vi "Evaluate Menu Selection.vi"(8 "error in":errorcluster, 9 "ItemPath":string, 10 "ItemTag":string, 11 "MQ in":refnum<class "Delacor_lib_QMH_Message Queue.lvclass">) -> (0 "error out":errorcluster)   [LabVIEW 2022 SP3, in "UI Manager.lvlib"]
doc: "____\nHAMPEL SOFTWARE ENGINEERING v2.6.0 (2023-12-19 10:54)"
uses:
  UI Manager.lvlib
  <vilib>/Delacor/Delacor QMH/Libraries/Message Queue_class/Delacor_lib_QMH_Message Queue.lvclass
  Shutdown Application Argument--cluster.ctl
  <vilib>/Delacor/Delacor QMH/Libraries/Message Queue_class/Delacor_lib_QMH_Message Queue.lvclass/Delacor_lib_QMH_Message Queue.ctl
  Display another Module UI Argument--cluster.ctl
  Module Display Scenarios.ctl
  Libraries/hse-libraries/Source/hse-application/hse-application.lvclass/hse-application.ctl
  <vilib>/Delacor/Delacor QMH/Libraries/Message Queue_class/Delacor_lib_QMH_Enqueue Message (Single).vi
  Libraries/hse-libraries/Source/hse-application/HSE Application not initialized--error.vi
  <vilib>/Utility/error.llb/Clear Errors.vi
  Libraries/hse-libraries/Source/hse-application/hse-application__GetSingleton.vi
  <vilib>/Utility/sysdir.llb/Get System Directory.vi
  <vilib>/Utility/error.llb/Error Cluster From Error Code.vi
  Libraries/hse-libraries/Source/hse-application/hse-application.lvclass
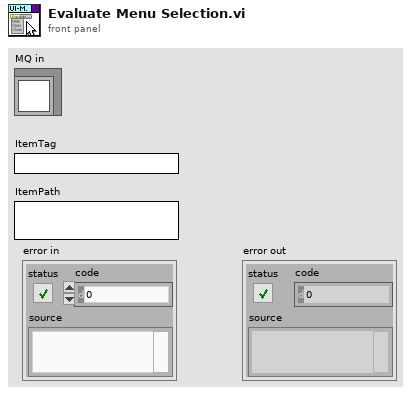
[diagram p1: front panel]
types:
  T1 = typedef "UI Manager.lvlib/Shutdown Application Argument--cluster.ctl" = cluster{"User Confirm?":bool}
  T2 = typedef "UI Manager.lvlib/Module Display Scenarios.ctl" = enum16{"Stand-Alone", "Managed"}
  T3 = typedef "UI Manager.lvlib/Display another Module UI Argument--cluster.ctl" = cluster{"Module DQMH Path":path, "Display Scenario":T2}
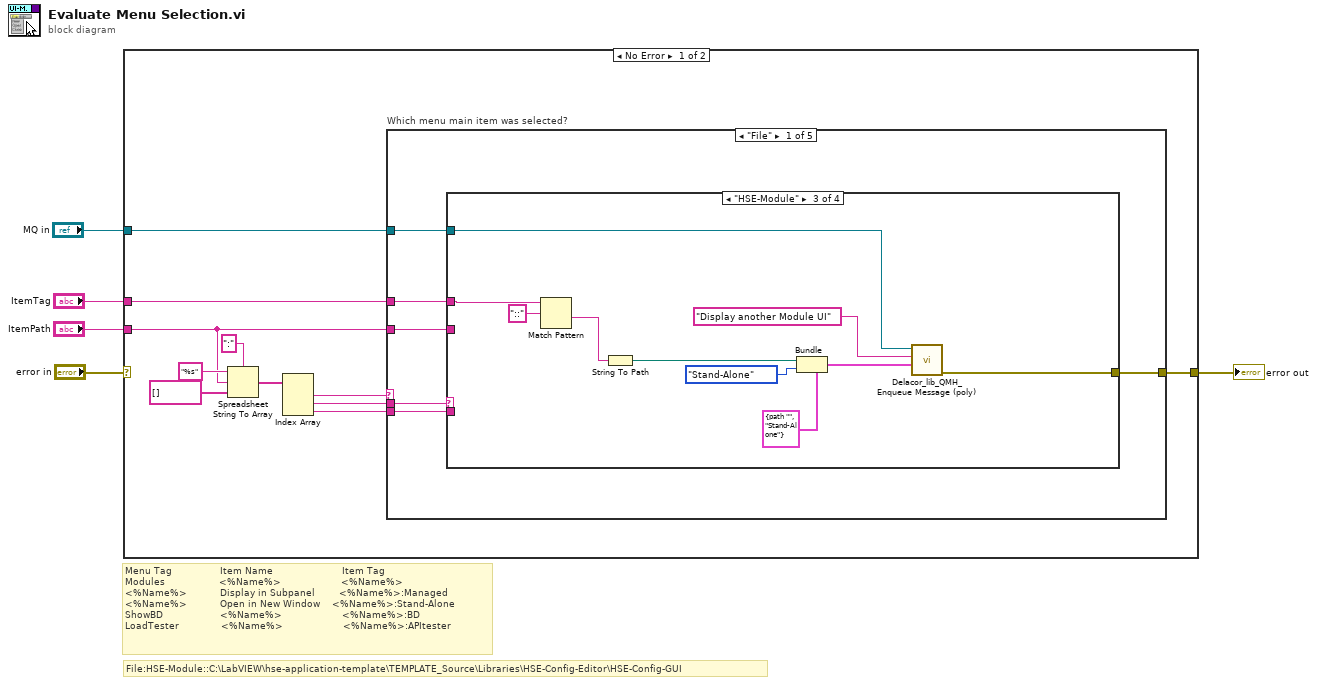
[diagram p0: block diagram]
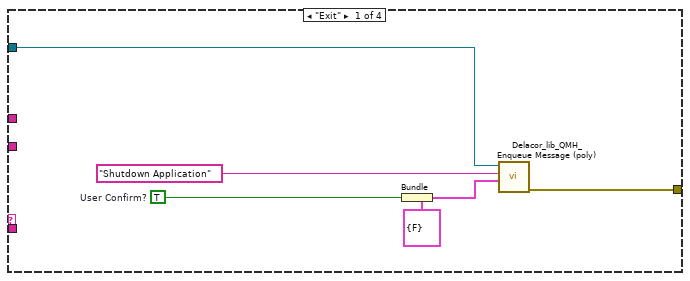
[diagram p2: hidden frame]
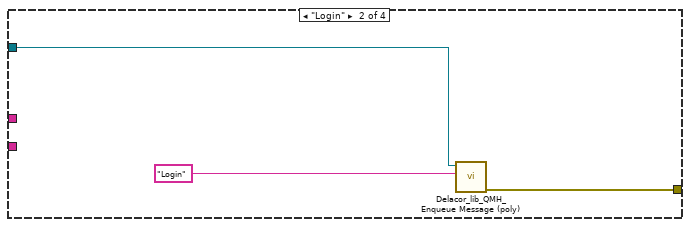
[diagram p3: hidden frame]
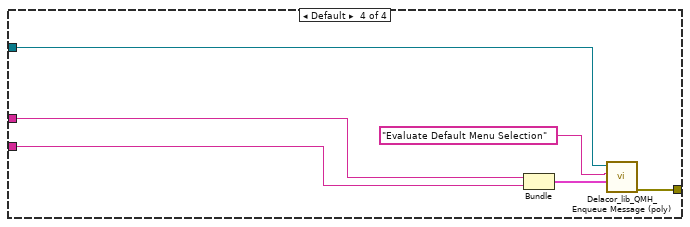
[diagram p4: hidden frame]
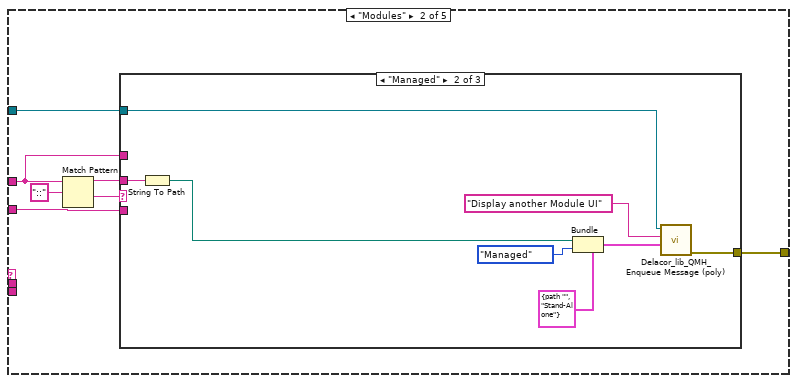
[diagram p5: hidden frame]
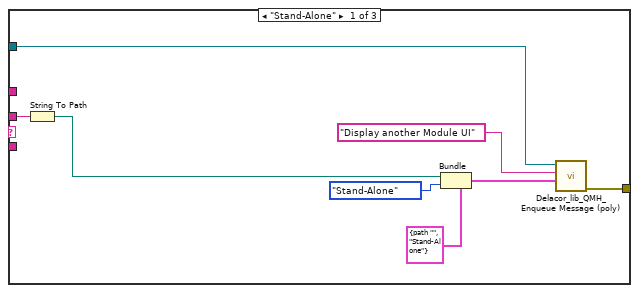
[diagram p6: hidden frame]
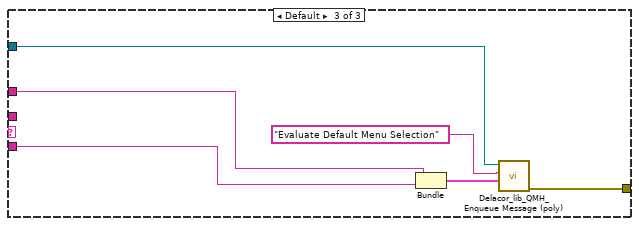
[diagram p7: hidden frame]
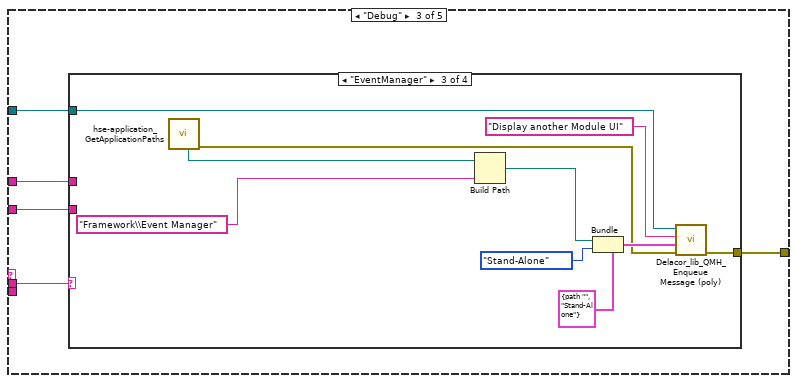
[diagram p8: hidden frame]
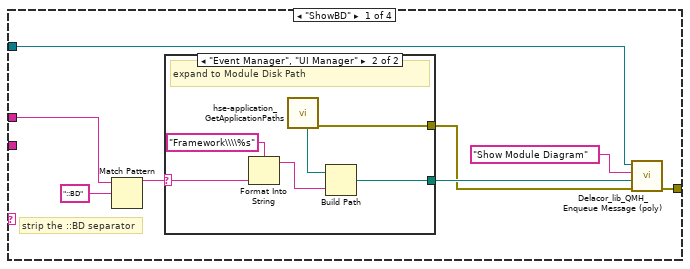
[diagram p9: hidden frame]
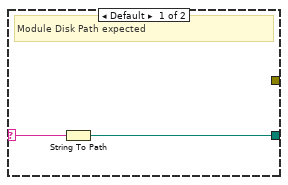
[diagram p10: hidden frame]
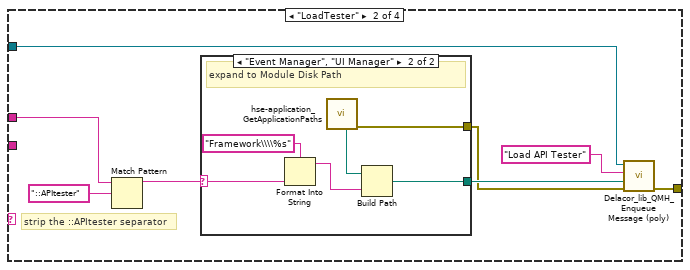
[diagram p11: hidden frame]
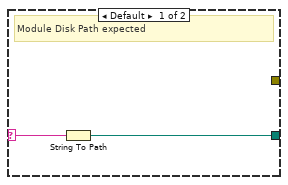
[diagram p12: hidden frame]
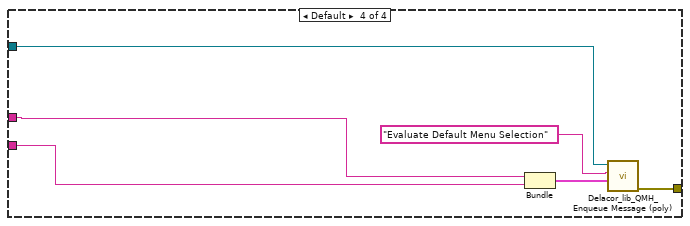
[diagram p13: hidden frame]
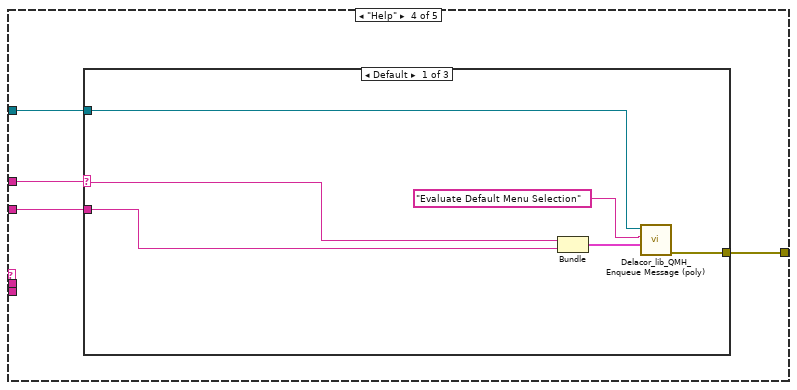
[diagram p14: hidden frame]
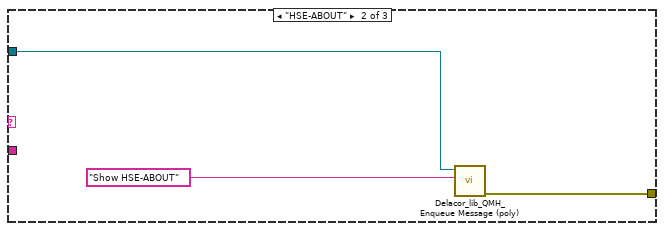
[diagram p15: hidden frame]
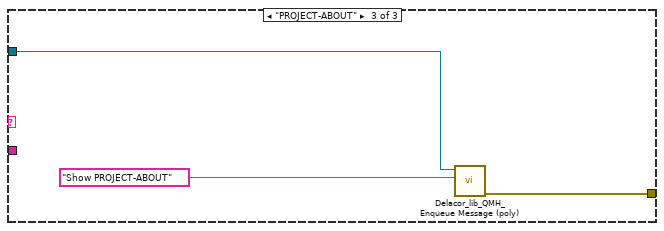
[diagram p16: hidden frame]
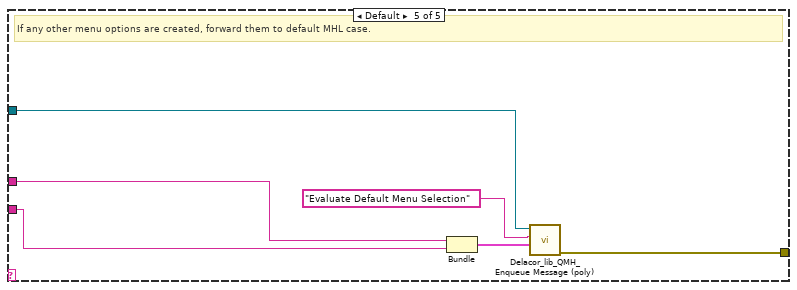
[diagram p17: hidden frame]
diagram:
  # "File:HSE-Module::C:\\LabVIEW\\hse-application-template\\TEMPLATE_Source\\Libraries\\HSE-Config-Editor\\HSE-Config-GUI"
  # "Menu Tag                Item Name\t                      Item Tag\nModules\t                 <%Name%>                   \t<%Name%>\n<%Name%>          \tDisplay in Subpanel       \t<%Name%>:Managed\n<%Name%>          \tOpen in New Window   \t<%Name%>:Stand-Alone\nShowBD                   <%Name%>\t                   <%Name%>:BD\nLoadTester\t             <%Name%>                   \t<%Name%>:APItester"
  n1 = case shown="No Error" "error in" {
    selector: "error in" -> [_ w152]
    tunnel: "ItemPath" -> [w6 _]
    tunnel: "MQ in" -> [w14 _]
    tunnel: "ItemTag" -> [w13 _]
    tunnel: [w11 w152] -> w2
    frame No Error {
      n2 = Spreadsheet String To Array(delimiter (Tab)=":", format string="%s", spreadsheet string=w6, array type (2D Dbl)=string[] []) -> (array=w10:string[])
      n3 = Index Array(array=w10) -> (element #1=w9:string, element #2=w7:string, element #3=w8:string)  [unwired: 3 in]
      n4 = case "Which menu main item was selected?" shown="\"File\"" w9 {
        tunnel: w14 -> [w22 w54 w81 w133 w151]
        tunnel: [w21 w53 w79 w132 w150] -> w11
        tunnel: w13 -> [w20 w49 w80 w131 w149]
        tunnel: w8 -> [w17 _ _ _ _]
        tunnel: w7 -> [w18 _ w78 _ _]
        tunnel: w6 -> [w19 w48 w77 w130 w146]
        frame "File" {
          n5 = case shown="\"HSE-Module\"" w18 {
            tunnel: w22 -> [w27 w30 w36 w44]
            tunnel: [w26 w29 w35 w45] -> w21
            tunnel: w19 -> [_ _ _ w42]
            tunnel: w20 -> [_ _ w33 w43]
            tunnel: w17 -> [_ _ _ _]
            frame "Exit" {
              w24 = TRUE  # User Confirm?
              n6 = Bundle(cluster=T1 {"User Confirm?"=FALSE} ("Shutdown Application Argument"), "User Confirm?"=w24) -> (w23:T1)
              n7 = call-poly <vilib>:"Delacor_lib_QMH_Enqueue Message (poly).vi"("Message Data"=w23, "Message"="Shutdown Application", "Message Queue in"=w27) -> ("error out"=w26:errorcluster)  [unwired: 7 in, 1 out]
            }
            frame "Login" {
              n8 = call-poly <vilib>:"Delacor_lib_QMH_Enqueue Message (poly).vi"("Message"="Login", "Message Queue in"=w30) -> ("error out"=w29:errorcluster)  [unwired: 8 in, 1 out]
            }
            frame "HSE-Module" {
              n9 = Match Pattern(string=w33, regular expression="::") -> (after substring=w32:string)  [unwired: 1 in, 3 out]
              n10 = String To Path(string=w32) -> (path=w41:path)
              n11 = Bundle(cluster=T3 {"Module DQMH Path"=path "", "Display Scenario"=enum."Stand-Alone"} ("Display Module UI Argument"), "Module DQMH Path"=w41, "Display Scenario"=Module_Display_Scenarios."Stand-Alone") -> (w38:T3)
              n12 = call-poly <vilib>:"Delacor_lib_QMH_Enqueue Message (poly).vi"("Message Data"=w38, "Message"="Display another Module UI", "Message Queue in"=w36) -> ("error out"=w35:errorcluster)  [unwired: 7 in, 1 out]
            }
            frame Default {
              n13 = Bundle("ItemTag"=w43, "ItemPath"=w42) -> (w46:cluster{"ItemTag":string, "ItemPath":string})  [unwired: 1 in]
              n14 = call-poly <vilib>:"Delacor_lib_QMH_Enqueue Message (poly).vi"("Message Data"=w46, "Message"="Evaluate Default Menu Selection", "Message Queue in"=w44) -> ("error out"=w45:errorcluster)  [unwired: 7 in, 1 out]
            }
          }
        }
        frame "Modules" {
          n15 = Match Pattern(string=w49, regular expression="::") -> (before substring=w50:string, after substring=w51:string)  [unwired: 1 in, 2 out]
          n16 = case shown="\"Managed\"" w51 {
            tunnel: w54 -> [w61 w65 w74]
            tunnel: [w57 w66 w73] -> w53
            tunnel: w50 -> [w56 w64 _]
            tunnel: w49 -> [_ _ w72]
            tunnel: w48 -> [_ _ w71]
            frame "Stand-Alone" {
              n17 = String To Path(string=w56) -> (path=w55:path)
              n18 = Bundle(cluster=T3 {"Module DQMH Path"=path "", "Display Scenario"=enum."Stand-Alone"} ("Display Module UI Argument"), "Module DQMH Path"=w55, "Display Scenario"=Module_Display_Scenarios."Stand-Alone") -> (w59:T3)
              n19 = call-poly <vilib>:"Delacor_lib_QMH_Enqueue Message (poly).vi"("Message Data"=w59, "Message"="Display another Module UI", "Message Queue in"=w61) -> ("error out"=w57:errorcluster)  [unwired: 7 in, 1 out]
            }
            frame "Managed" {
              n20 = String To Path(string=w64) -> (path=w63:path)
              n21 = Bundle(cluster=T3 {"Module DQMH Path"=path "", "Display Scenario"=enum."Stand-Alone"} ("Display Module UI Argument"), "Module DQMH Path"=w63, "Display Scenario"=Module_Display_Scenarios."Managed") -> (w68:T3)
              n22 = call-poly <vilib>:"Delacor_lib_QMH_Enqueue Message (poly).vi"("Message Data"=w68, "Message"="Display another Module UI", "Message Queue in"=w65) -> ("error out"=w66:errorcluster)  [unwired: 7 in, 1 out]
            }
            frame Default {
              n23 = Bundle("ItemTag"=w72, "ItemPath"=w71) -> (w75:cluster{"ItemTag":string, "ItemPath":string})  [unwired: 1 in]
              n24 = call-poly <vilib>:"Delacor_lib_QMH_Enqueue Message (poly).vi"("Message Data"=w75, "Message"="Evaluate Default Menu Selection", "Message Queue in"=w74) -> ("error out"=w73:errorcluster)  [unwired: 7 in, 1 out]
            }
          }
        }
        frame "Debug" {
          n25 = case shown="\"EventManager\"" w78 {
            tunnel: w81 -> [w88 w104 w118 w126]
            tunnel: w80 -> [w85 w101 _ w125]
            tunnel: [w87 w103 w119 w127] -> w79
            tunnel: w77 -> [_ _ _ w124]
            frame "ShowBD" {
              # "strip the ::BD separator"
              n26 = Match Pattern(string=w85, regular expression="::BD") -> (before substring=w84:string)  [unwired: 1 in, 3 out]
              n27 = case shown="\"Event Manager\", \"UI Manager\"" w84 {
                selector: w84 -> [w91 w96]
                tunnel: [w90 w94] -> w83
                tunnel: [_ w93] -> w82
                frame Default {
                  # "Module Disk Path expected"
                  n28 = String To Path(string=w91) -> (path=w90:path)
                }
                frame "Event Manager", "UI Manager" {
                  # "expand to Module Disk Path"
                  n29 = Format Into String(format string="Framework\\\\%s" ("Module Name"), w96) -> (resulting string=w95:string)  [unwired: 2 in, 1 out]
                  n30 = call "hse-application_GetApplicationPaths.vi"() -> ("error out"=w93:errorcluster, "Application Base Path"=w92:path)  [unwired: 5 in, 5 out]
                  n31 = Build Path(base path=w92, name or relative path=w95) -> (appended path=w94:path)
                }
              }
              n32 = call-poly <vilib>:"Delacor_lib_QMH_Enqueue Message (poly).vi"("error in"=w82, "Message Data"=w83, "Message"="Show Module Diagram", "Message Queue in"=w88) -> ("error out"=w87:errorcluster)  [unwired: 6 in, 1 out]
            }
            frame "LoadTester" {
              # "strip the ::APItester separator"
              n33 = Match Pattern(string=w101, regular expression="::APItester") -> (before substring=w100:string)  [unwired: 1 in, 3 out]
              n34 = case shown="\"Event Manager\", \"UI Manager\"" w100 {
                selector: w100 -> [w107 w112]
                tunnel: [w106 w110] -> w99
                tunnel: [_ w109] -> w98
                frame Default {
                  # "Module Disk Path expected"
                  n35 = String To Path(string=w107) -> (path=w106:path)
                }
                frame "Event Manager", "UI Manager" {
                  # "expand to Module Disk Path"
                  n36 = Format Into String(format string="Framework\\\\%s" ("Module Name"), w112) -> (resulting string=w111:string)  [unwired: 2 in, 1 out]
                  n37 = call "hse-application_GetApplicationPaths.vi"() -> ("error out"=w109:errorcluster, "Application Base Path"=w108:path)  [unwired: 5 in, 5 out]
                  n38 = Build Path(base path=w108, name or relative path=w111) -> (appended path=w110:path)
                }
              }
              n39 = call-poly <vilib>:"Delacor_lib_QMH_Enqueue Message (poly).vi"("error in"=w98, "Message Data"=w99, "Message"="Load API Tester", "Message Queue in"=w104) -> ("error out"=w103:errorcluster)  [unwired: 6 in, 1 out]
            }
            frame "EventManager" {
              n40 = call "hse-application_GetApplicationPaths.vi"() -> ("error out"=w114:errorcluster, "Application Base Path"=w115:path)  [unwired: 5 in, 5 out]
              n41 = Build Path(base path=w115, name or relative path="Framework\\Event Manager" ("Module Name")) -> (appended path=w116:path)
              n42 = Bundle(cluster=T3 {"Module DQMH Path"=path "", "Display Scenario"=enum."Stand-Alone"} ("Display Module UI Argument"), "Module DQMH Path"=w116, "Display Scenario"=Module_Display_Scenarios."Stand-Alone") -> (w121:T3)
              n43 = call-poly <vilib>:"Delacor_lib_QMH_Enqueue Message (poly).vi"("error in"=w114, "Message Data"=w121, "Message"="Display another Module UI", "Message Queue in"=w118) -> ("error out"=w119:errorcluster)  [unwired: 6 in, 1 out]
            }
            frame Default {
              n44 = Bundle("ItemTag"=w125, "ItemPath"=w124) -> (w128:cluster{"ItemTag":string, "ItemPath":string})  [unwired: 1 in]
              n45 = call-poly <vilib>:"Delacor_lib_QMH_Enqueue Message (poly).vi"("Message Data"=w128, "Message"="Evaluate Default Menu Selection", "Message Queue in"=w126) -> ("error out"=w127:errorcluster)  [unwired: 7 in, 1 out]
            }
          }
        }
        frame "Help" {
          n46 = case shown="Default" w131 {
            selector: w131 -> [w135 _ _]
            tunnel: w133 -> [w136 w142 w145]
            tunnel: [w137 w140 w143] -> w132
            tunnel: w130 -> [w134 _ _]
            frame Default {
              n47 = Bundle(w135, "ItemPath"=w134) -> (w138:cluster{string, "ItemPath":string})  [unwired: 1 in]
              n48 = call-poly <vilib>:"Delacor_lib_QMH_Enqueue Message (poly).vi"("Message Data"=w138, "Message"="Evaluate Default Menu Selection", "Message Queue in"=w136) -> ("error out"=w137:errorcluster)  [unwired: 7 in, 1 out]
            }
            frame "HSE-ABOUT" {
              n49 = call-poly <vilib>:"Delacor_lib_QMH_Enqueue Message (poly).vi"("Message"="Show HSE-ABOUT", "Message Queue in"=w142) -> ("error out"=w140:errorcluster)  [unwired: 8 in, 1 out]
            }
            frame "PROJECT-ABOUT" {
              n50 = call-poly <vilib>:"Delacor_lib_QMH_Enqueue Message (poly).vi"("Message"="Show PROJECT-ABOUT", "Message Queue in"=w145) -> ("error out"=w143:errorcluster)  [unwired: 8 in, 1 out]
            }
          }
        }
        frame Default {
          # "If any other menu options are created, forward them to default MHL case."
          n51 = Bundle("ItemTag"=w149, "ItemPath"=w146) -> (w147:cluster{"ItemTag":string, "ItemPath":string})  [unwired: 1 in]
          n52 = call-poly <vilib>:"Delacor_lib_QMH_Enqueue Message (poly).vi"("Message Data"=w147, "Message"="Evaluate Default Menu Selection", "Message Queue in"=w151) -> ("error out"=w150:errorcluster)  [unwired: 7 in, 1 out]
        }
      }
    }
    frame Error {
    }
  }
  "error out" <- w2
